vi "DefaultFromIni.vi"(8 "error in (no error)":errorcluster, 11 "SiemensDigitalEnergyMeter in":refnum<class "SiemensDigitalEnergyMeter.lvclass">) -> (0 "error out":errorcluster, 3 "SiemensDigitalEnergyMeter out":refnum<class "SiemensDigitalEnergyMeter.lvclass">)   [LabVIEW 2018, in "SensorPlugins.lvlib" / "SiemensDigitalEnergyMeter.lvclass"]
doc: "This VI opens the configuration INI file and loads the information from the file into the class cluster."
uses:
  SiemensDigitalEnergyMeter.lvclass
  C:/Program Files (x86)/National Instruments/LabVIEW 2018/user.lib/NIST/BaseClasses/BasePlugin_class/BasePlugin.lvclass
  TypeDefinitions/SiemensDigitalEnergyMeterControls.ctl
  <userlib>/NIST/BaseClasses/BasePlugin_class/BasePlugin.lvclass/BasePlugin.ctl
  TypeDefinitions/MeasurementControls.ctl
  <userlib>/NIST/BaseClasses/BasePlugin_class/Accessors/Read PluginIniFilePath.vi
  <vilib>/Utility/error.llb/Error Cluster From Error Code.vi
  <vilib>/ErrorRing/Error Ring.xnode
  <vilib>/Utility/config.llb/NI_LVConfig.lvlib
  TestClass/Test.lvclass
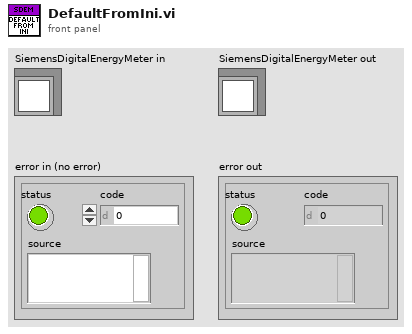
[diagram p1: front panel]
types:
  T1 = typedef "SensorPlugins.lvlib/SiemensDigitalEnergyMeter.lvclass/MeasurementControls.ctl" = cluster{"Measurement RefreshTime (ms)":u32, "Measurement Name":string}
  T2 = typedef "SensorPlugins.lvlib/SiemensDigitalEnergyMeter.lvclass/SiemensDigitalEnergyMeterControls.ctl" = cluster{"Measurement(s)":u16[], "Configuration Commands":string, "Use Measurement Commands Text Box?":bool, "Measurement Commands":string, "Connected?":bool, "Serial Number":string, "IP Address":string, "Port (502)":u16, "Unit ID":u8, "Serial Type":enum16{"RTU", "ASCII"}, "Using TCP?":bool, "VISA Resource Name":string}[]
  T3 = typedef "NI_LVConfig.lvlib/Config Data RefNum.ctl" = refnum<k1>
  T4 = typedef "Test.lvclass/INIInfo.ctl" = cluster{"Module Name":string, "INI File Name":string, "Class Name":string, "INI File Name Without Extension":string, "Module.Class.INI File Name":string, "Visualization VI Path":path, "Instrument Class Path":path}
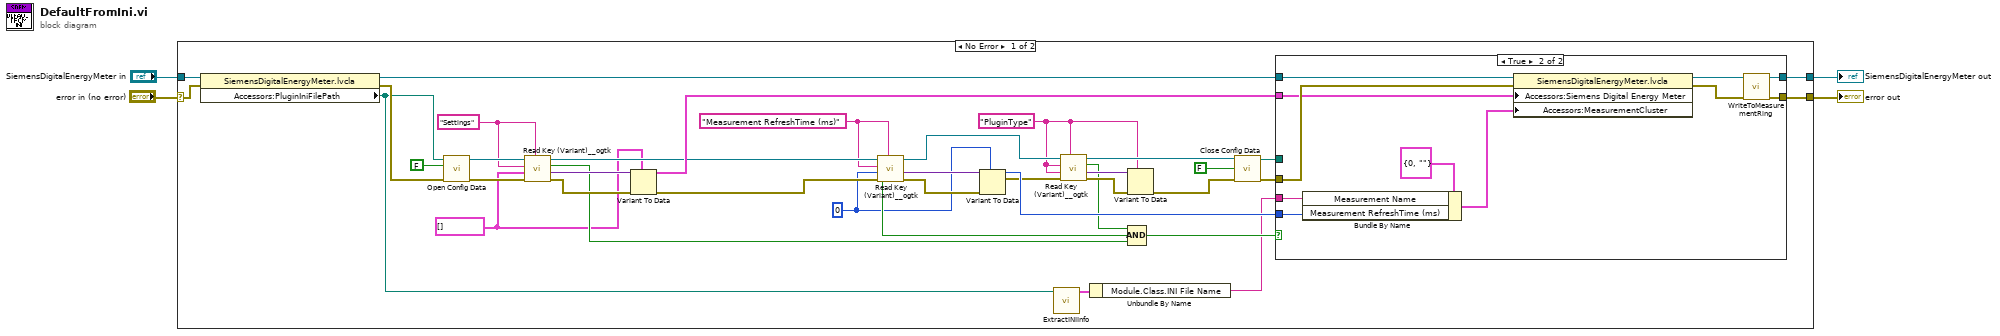
[diagram p0: block diagram]
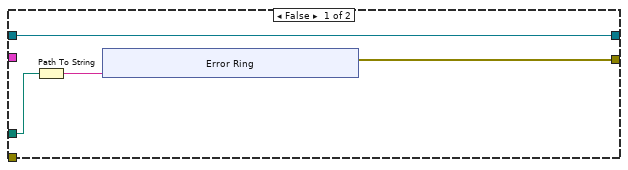
[diagram p2: hidden frame]
diagram:
  n1 = case shown="No Error" "error in (no error)" {
    selector: "error in (no error)" -> [w41 w65]
    tunnel: "SiemensDigitalEnergyMeter in" -> [w42 w66]
    tunnel: [w35 w66] -> w2
    tunnel: [w31 w65] -> w1
    frame No Error {
      w8 = "PluginType" ("section")
      w16 = u32 0 ("Measurement RefreshTime (ms)")
      w17 = T2 [] ("Siemens Digital Energy Meter")
      w19 = "Measurement RefreshTime (ms)" ("section")
      w28 = "Settings" ("section")
      n2 = property class="SiemensDigitalEnergyMeter.lvcla"(reference=w42, error in=w41) -> (reference out=w36:refnum<class "SiemensDigitalEnergyMeter.lvclass">, error out=w39:errorcluster, "Accessors:PluginIniFilePath"=w7:path)
      n3 = call <vilib>:"Open Config Data.vi"("error in (no error)"=w39, "create file if necessary (T)"=FALSE, "configuration file path"=w7) -> ("error out"=w37:errorcluster, "refnum"=w38:T3)  [unwired: 6 in, 1 out]
      n4 = call <userlib>:"Read Key (Variant)__ogtk.vi"("section"=w28, "error in (no error)"=w37, "type"=w17, "key (optional)"=w28, "refnum"=w38) -> ("error out"=w33:errorcluster, "key-value"=w34:variant, "found?"=w26:bool, "refnum out"=w21:T3)  [unwired: 3 in]
      n5 = Variant To Data(error in=w33, type=w17, Variant=w34) -> (data=w32:T2, error out=w22:errorcluster)
      n6 = call <userlib>:"Read Key (Variant)__ogtk.vi"("section"=w19, "error in (no error)"=w22, "type"=w16, "key (optional)"=w19, "refnum"=w21) -> ("error out"=w24:errorcluster, "key-value"=w23:variant, "found?"=w20:bool, "refnum out"=w14:T3)  [unwired: 3 in]
      n7 = Variant To Data(error in=w24, type=w16, Variant=w23) -> (data=w18:u32, error out=w15:errorcluster)
      n8 = call "ExtractINIInfo.vi"("INI File Path"=w7) -> ("INI Info"=w6:T4)  [unwired: 4 in, 6 out]
      n9 = call <userlib>:"Read Key (Variant)__ogtk.vi"("section"=w8, "error in (no error)"=w15, "type"=w8, "key (optional)"=w8, "refnum"=w14) -> ("error out"=w12:errorcluster, "key-value"=w10:variant, "found?"=w9:bool, "refnum out"=w13:T3)  [unwired: 3 in]
      n10 = Unbundle By Name(w6) -> ("Module.Class.INI File Name"=w5:string)
      n11 = Variant To Data(error in=w12, type=w8, Variant=w10) -> (error out=w11:errorcluster)  [unwired: 1 out]
      n12 = Compound Arithmetic op=AND(w9, w20, w26) -> (w27:bool)
      n13 = call <vilib>:"Close Config Data.vi"("error in (no error)"=w11, "write file if changed (T)"=FALSE, "refnum"=w13) -> ("error out"=w30:errorcluster, "file path"=w25:path)  [unwired: 7 in]
      n14 = case shown="True" w27 {
        tunnel: w36 -> [w46 w64]
        tunnel: [w46 w58] -> w35
        tunnel: w32 -> [_ w62]
        tunnel: [w43 w60] -> w31
        tunnel: w30 -> [_ w63]
        tunnel: w25 -> [w44 _]
        tunnel: w18 -> [_ w56]
        tunnel: w5 -> [_ w55]
        frame False {
          n15 = Path To String(path=w44) -> (string=w45:string)
          n16 = xnode "Error Ring"("parameter 0"=w45) -> ("error out"=w43:errorcluster)
        }
        frame True {
          n17 = Bundle By Name(cluster=T1 {"Measurement RefreshTime (ms)"=0, "Measurement Name"=""} ("MeasurementCluster"), "Measurement Name"=w55, "Measurement RefreshTime (ms)"=w56) -> (w54:T1)
          n18 = property class="SiemensDigitalEnergyMeter.lvcla"(reference=w64, error in=w63, "Accessors:Siemens Digital Energy Meter"=w62, "Accessors:MeasurementCluster"=w54) -> (reference out=w59:refnum<class "SiemensDigitalEnergyMeter.lvclass">, error out=w61:errorcluster)
          n19 = call-dynamic "WriteToMeasurementRing.vi"("error in (no error)"=w61, "SiemensDigitalEnergyMeter in"=w59) -> ("error out"=w60:errorcluster, "SiemensDigitalEnergyMeter out"=w58:refnum<class "SiemensDigitalEnergyMeter.lvclass">)  [unwired: 8 in]
        }
      }
    }
    frame Error {
    }
  }
  "error out" <- w1
  "SiemensDigitalEnergyMeter out" <- w2
